vi "DomainMetadata.FGV.vi"(7 "Case Select":T2(ring), 8 "error in":errorcluster, 9 "Int in":i64, 10 "String in":string, 11 "DomainMetadata in":T1) -> (0 "error out":errorcluster, 3 "DomainMetadata out":T1)   [LabVIEW 2022 SP3, in "openDAQ.lvlib" / "daqUtils.lvlib"]
uses:
  <instrlib>/openDAQ/Public/Classes/daqUtils/daqUtils.lvlib
  <instrlib>/openDAQ/Public/TypeDef/DomainMetadata.ctl
  <instrlib>/openDAQ/openDAQ.lvlib
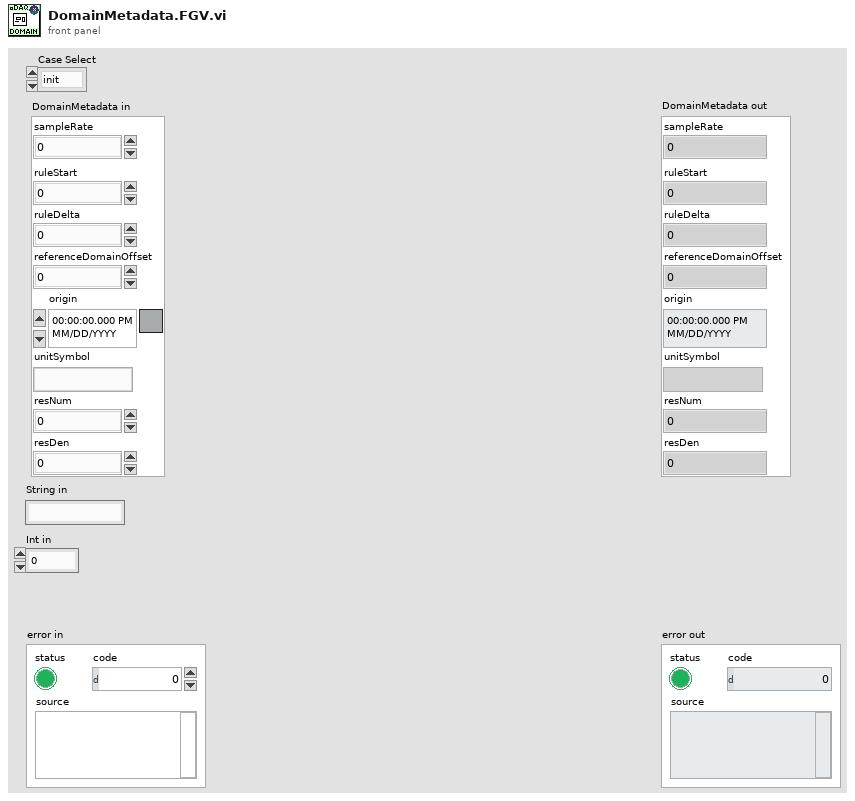
[diagram p1: front panel]
types:
  T1 = typedef "openDAQ.lvlib/DomainMetadata.ctl" = cluster{"sampleRate":i64, "ruleStart":i64, "ruleDelta":i64, "referenceDomainOffset":i64, "origin":timestamp, "unitSymbol":string, "resNum":i64, "resDen":i64}
  T2 = enum16{"init", "read", "set sampleRate", "set ruleStart", "set ruleDelta", "set referenceDomainOffset", "set origin", "set unitSymbol", "set resNum", "set resDen", " calculate sampleRate"}
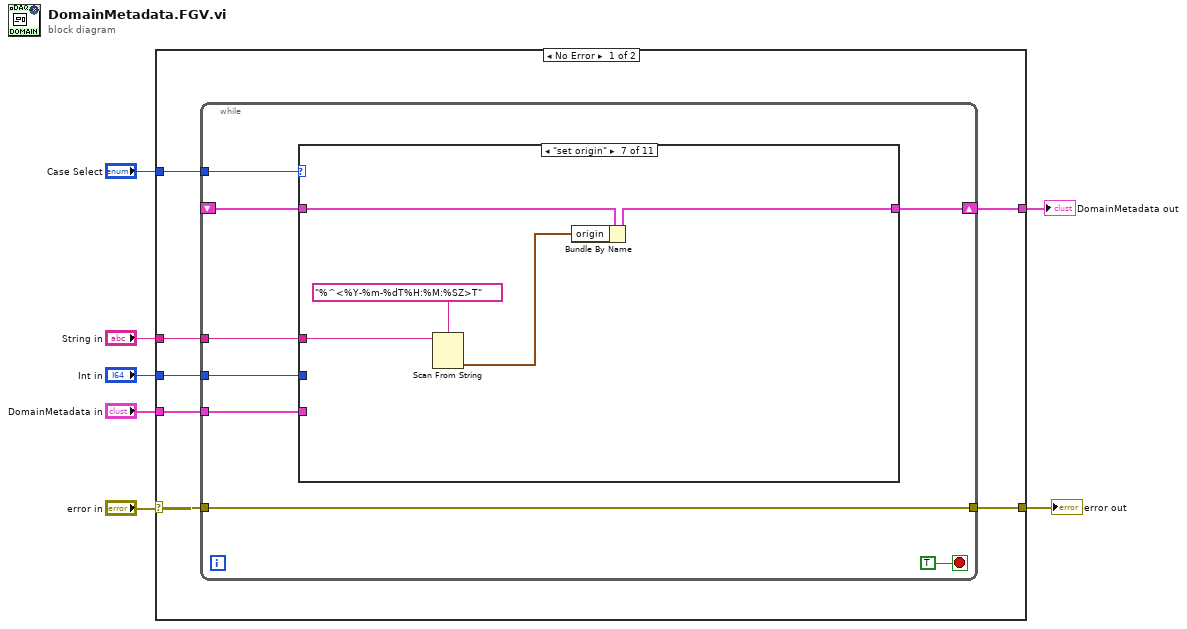
[diagram p0: block diagram]
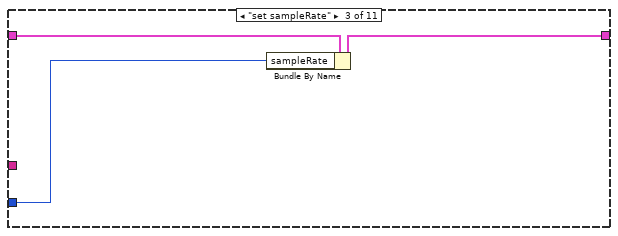
[diagram p4: hidden frame]
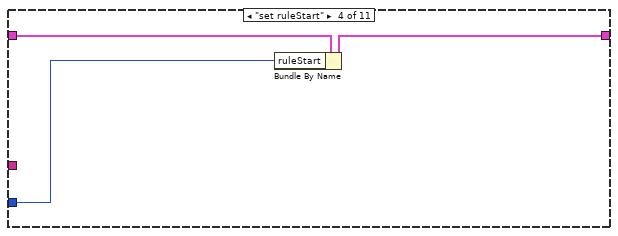
[diagram p5: hidden frame]
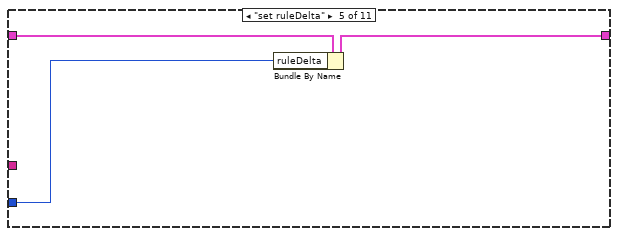
[diagram p6: hidden frame]
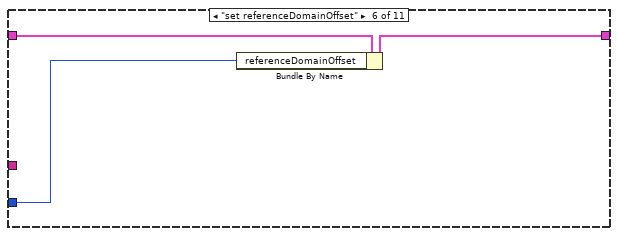
[diagram p7: hidden frame]
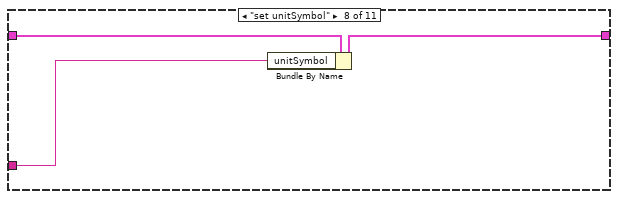
[diagram p8: hidden frame]
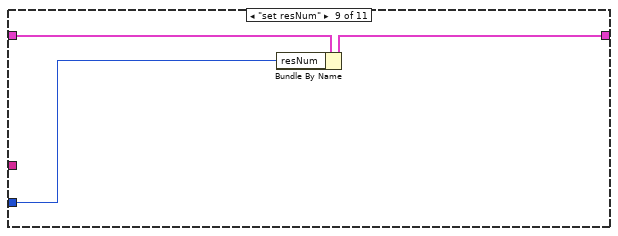
[diagram p9: hidden frame]
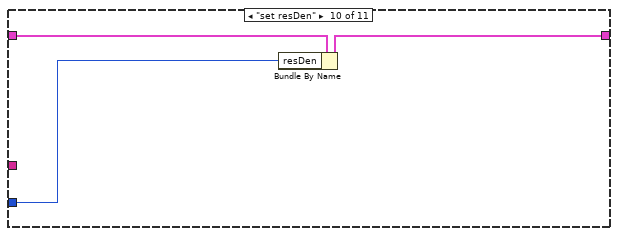
[diagram p10: hidden frame]
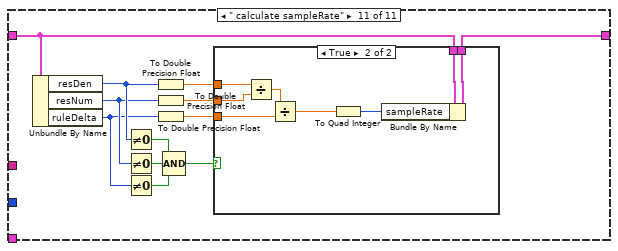
[diagram p11: hidden frame]
diagram:
  n1 = case shown="No Error" "error in" {
    selector: "error in" -> [w14 w72]
    tunnel: [w13 w72] -> w6
    tunnel: "Case Select" -> [w12 _]
    tunnel: "DomainMetadata in" -> [w11 _]
    tunnel: [w10 _] -> w3
    tunnel: "String in" -> [w9 _]
    tunnel: "Int in" -> [w8 _]
    frame No Error {
      n2 = while {
        tunnel: w14 -> [w22]
        tunnel: [w22] -> w13
        tunnel: w12 -> [w20]
        tunnel: w11 -> [w19]
        shift-right: [w18] -> w10
        shift-left: _ -> [w17]
        tunnel: w9 -> [w16]
        tunnel: w8 -> [w15]
        stop <- TRUE stop-if-true
        n3 = case shown="\"set origin\"" w20 {
          tunnel: w19 -> [w23 _ _ _ _ _ _ _ _ _ _]
          tunnel: [w23 w24 w26 w29 w32 w35 w40 w43 w46 w49 w58] -> w18
          tunnel: w17 -> [_ w24 w27 w30 w33 w36 w41 w44 w47 w50 w59]
          tunnel: w16 -> [_ _ _ _ _ _ w39 w42 _ _ _]
          tunnel: w15 -> [_ _ w25 w28 w31 w34 _ _ w45 w48 _]
          frame "init" {
          }
          frame "read" {
          }
          frame "set sampleRate" {
            n4 = Bundle By Name(cluster=w27, "sampleRate"=w25) -> (w26:T1)
          }
          frame "set ruleStart" {
            n5 = Bundle By Name(cluster=w30, "ruleStart"=w28) -> (w29:T1)
          }
          frame "set ruleDelta" {
            n6 = Bundle By Name(cluster=w33, "ruleDelta"=w31) -> (w32:T1)
          }
          frame "set referenceDomainOffset" {
            n7 = Bundle By Name(cluster=w36, "referenceDomainOffset"=w34) -> (w35:T1)
          }
          frame "set origin" {
            n8 = Scan From String(format string="%^<%Y-%m-%dT%H:%M:%SZ>T", input string=w39) -> (output 1=w37:timestamp)  [unwired: 3 in, 3 out]
            n9 = Bundle By Name(cluster=w41, "origin"=w37) -> (w40:T1)
          }
          frame "set unitSymbol" {
            n10 = Bundle By Name(cluster=w44, "unitSymbol"=w42) -> (w43:T1)
          }
          frame "set resNum" {
            n11 = Bundle By Name(cluster=w47, "resNum"=w45) -> (w46:T1)
          }
          frame "set resDen" {
            n12 = Bundle By Name(cluster=w50, "resDen"=w48) -> (w49:T1)
          }
          frame " calculate sampleRate" {
            n13 = Unbundle By Name(w59) -> ("resDen"=w56:i64, "resNum"=w55:i64, "ruleDelta"=w54:i64)
            n14 = Not Equal To 0?(x=w56) -> (x != 0?=w62:bool)
            n15 = Not Equal To 0?(x=w55) -> (x != 0?=w61:bool)
            n16 = Not Equal To 0?(x=w54) -> (x != 0?=w60:bool)
            n17 = To Double Precision Float(number=w56) -> (double precision float=w53:dbl)
            n18 = To Double Precision Float(number=w55) -> (double precision float=w52:dbl)
            n19 = To Double Precision Float(number=w54) -> (double precision float=w51:dbl)
            n20 = Compound Arithmetic op=AND(w62, w61, w60) -> (w57:bool)
            n21 = case shown="True" w57 {
              tunnel: w59 -> [w63 w71]
              tunnel: [w63 w70] -> w58
              tunnel: w53 -> [_ w69]
              tunnel: w52 -> [_ w68]
              tunnel: w51 -> [_ w66]
              frame False {
              }
              frame True {
                n22 = Divide(x=w69, y=w68) -> (x/y=w67:dbl)
                n23 = Divide(x=w67, y=w66) -> (x/y=w65:dbl)
                n24 = To Quad Integer(1:w65) -> (0:w64:i64)
                n25 = Bundle By Name(cluster=w71, "sampleRate"=w64) -> (w70:T1)
              }
            }
          }
        }
      }
    }
    frame Error {
    }
  }
  "error out" <- w6
  "DomainMetadata out" <- w3
